vi "CH_LM Transaction.vi"(0 "Meter Index":i32, 1 "Command String":string, 3 "NofStrings (-1:all)":i32=-1, 5 "error in (no error)":errorcluster, 7 "Timeout / ms (3000)":i32=10000, 9 "Lock Timeout / ms (1000)":i32=1000) -> (11 "Lock timed out":bool, 14 "Meter Index":i32, 15 "Response":string, 17 "Response Array":string[](array[string]), 19 "error out":errorcluster)   [LabVIEW 2017, in "CH_LM.lvlib"]
doc: "This VI is used by all other VI to communicate with a LabMax. It is designed as transaction to garantee that an instruments response belongs to the causing command. A semaphore is used to implement mutual exclusion of concurrent access to the communication interface. (The semaphore is created in the CH_LM ActiveX Control.vi.)"
uses:
  CH_LM.lvlib
  CH_LM Action Enumeration.ctl
  <vilib>/Utility/error.llb/DialogType.ctl
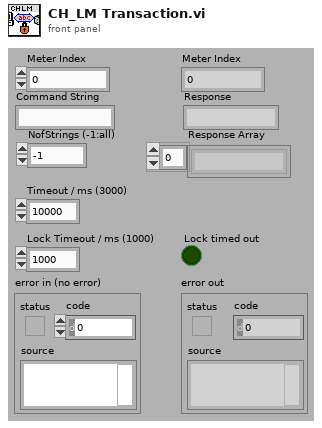
[diagram p1: front panel]
types:
  T1 = typedef "CH_LM.lvlib/CH_LM Action Enumeration.ctl" = enum16{"add", "read", "read by serial", "set", "remove", "delete", "Clear Shift-Register", ""}
  T2 = typedef "Semaphore RefNum" = refnum<k1>
  T3 = typedef "DialogType.ctl" = u16
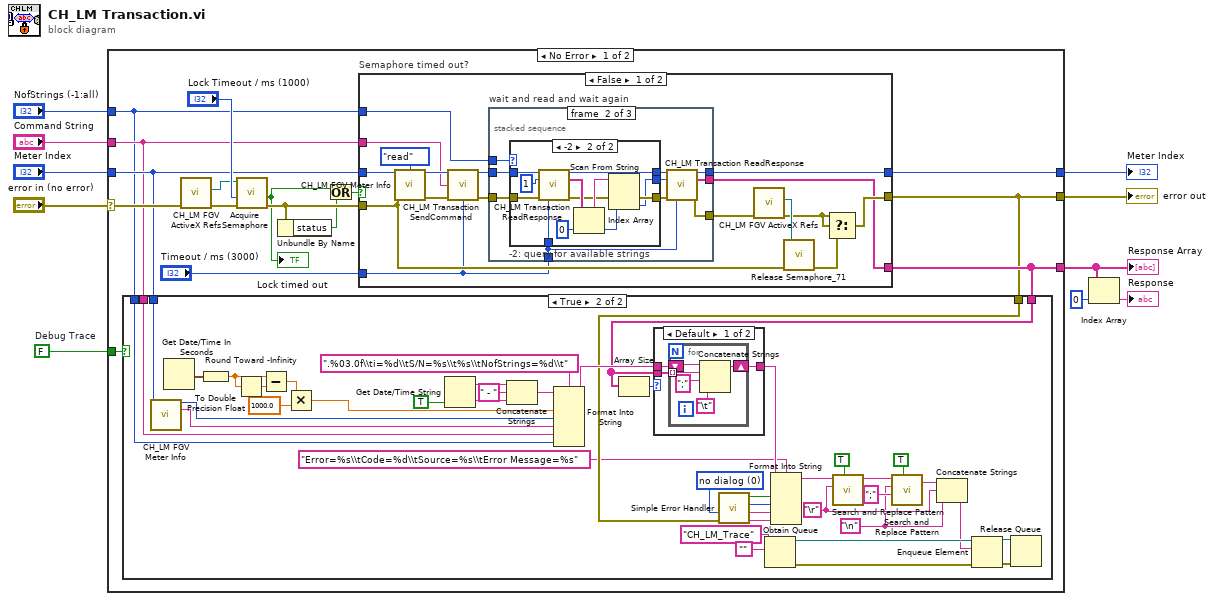
[diagram p0: block diagram]
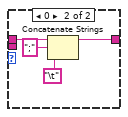
[diagram p3: hidden frame]
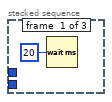
[diagram p4: hidden frame]
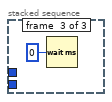
[diagram p6: hidden frame]
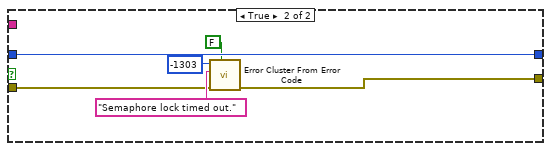
[diagram p7: hidden frame]
diagram:
  w1 = FALSE  # Debug Trace
  n1 = case shown="No Error" "error in (no error)" {
    selector: "error in (no error)" -> [w23 w132]
    tunnel: [w11 w132] -> w10
    tunnel: "Meter Index" -> [w15 w131]
    tunnel: [w12 _] -> w7
    tunnel: [w17 w131] -> w8
    tunnel: "Command String" -> [w14 _]
    tunnel: "NofStrings (-1:all)" -> [w13 _]
    tunnel: w1 -> [w16 _]
    frame No Error {
      n2 = call "CH_LM FGV ActiveX Refs.vi"("error in (no error)"=w23) -> ("error out"=w22:errorcluster, "CH_LM semaphore"=w24:T2)  [unwired: 4 in, 2 out]
      n3 = call <vilib>:"Acquire Semaphore.vi"("error in (no error)"=w22, "ms timeout (-1)"="Lock Timeout / ms (1000)", "semaphore"=w24) -> ("error out"=w21:errorcluster, "timed out"=w19:bool)  [unwired: 3 out]
      "Lock timed out" <- w19
      n4 = Unbundle By Name(w21) -> ("status"=w20:bool)
      n5 = Or(x=w19, y=w20) -> (x .or. y?=w18:bool)
      n6 = case "Semaphore timed out?" shown="False" w18 {
        tunnel: w14 -> [w92 _]
        tunnel: [w87 _] -> w12
        tunnel: [w98 w126] -> w11
        tunnel: "Timeout / ms (3000)" -> [w83 _]
        tunnel: w21 -> [w93 w127]
        tunnel: w15 -> [w95 w130]
        tunnel: w13 -> [w84 _]
        tunnel: [w88 w130] -> w17
        frame False {
          n7 = call "CH_LM FGV Meter Info.vi"("Meter Index"=w95, "Action (read)"=CH_LM_Action_Enumeration."read", "error in (no error)"=w93) -> ("Meter Index out"=w96:i32, "error out"=w94:errorcluster)  [unwired: 2 in, 9 out]
          n8 = call "CH_LM Transaction SendCommand.vi"("Meter Index"=w96, "Command String"=w92, "error in (no error)"=w94, "Timeout / ms (3000)"=w83) -> ("Meter Index out"=w85:i32, "error out"=w86:errorcluster)  [unwired: 4 in, 6 out]
          n9 = stacked-sequence "wait and read and wait again" {
            tunnel: [_ w109 _] -> w88
            tunnel: [_ w108 _] -> w87
            tunnel: w86 -> [_ w107 _]
            tunnel: w85 -> [_ w106 _]
            tunnel: w84 -> [_ w102 _]
            tunnel: w83 -> [_ w101 _]
            tunnel: [_ w100 _] -> w82
            frame #0 {
              n10 = Wait (ms)(milliseconds to wait=u32 20) -> ()  [unwired: 1 out]
            }
            frame #1 {
              n11 = case "-2: query for available strings" shown="-2" w102 {
                selector: w102 -> [w110 _]
                tunnel: w107 -> [w111 w123]
                tunnel: w106 -> [w112 w122]
                tunnel: [w112 w121] -> w105
                tunnel: [w111 w116] -> w104
                tunnel: [w110 w114] -> w103
                tunnel: w101 -> [_ w113]
                frame Default {
                }
                frame -2 {
                  w115 = 0 ("index")
                  n12 = call "CH_LM Transaction ReadResponse.vi"("Meter Index"=w122, "NofStrings (-1:all)"=1, "error in (no error)"=w123, "Timeout / ms (3000)"=w113) -> ("Meter Index out"=w121:i32, "Response Array"=w119:string[], "error out"=w117:errorcluster)  [unwired: 9 out]
                  n13 = Index Array(array=w119, index=w115) -> (element=w118:string)
                  n14 = Scan From String(input string=w118, error in=w117, default 1=w115) -> (error out=w116:errorcluster, output 1=w114:i32)  [unwired: 2 in, 2 out]
                }
              }
              n15 = call "CH_LM Transaction ReadResponse.vi"("Meter Index"=w105, "NofStrings (-1:all)"=w103, "error in (no error)"=w104, "Timeout / ms (3000)"=w101) -> ("Meter Index out"=w109:i32, "Response Array"=w108:string[], "error out"=w100:errorcluster)  [unwired: 9 out]
            }
            frame #2 {
              n16 = Wait (ms)(milliseconds to wait=u32 0) -> ()  [unwired: 1 out]
            }
          }
          n17 = call "CH_LM FGV ActiveX Refs.vi"("error in (no error)"=w82) -> ("error out"=w89:errorcluster, "CH_LM semaphore"=w90:T2)  [unwired: 4 in, 2 out]
          n18 = call <vilib>:"Release Semaphore_71.vi"("error in (no error)"=w93, "semaphore"=w90) -> ("error out"=w91:errorcluster)  [unwired: 5 out]
          n19 = Select(t=w89, s=w89, f=w91) -> (s? t:f=w98:errorcluster)
        }
        frame True {
          n20 = call <vilib>:"Error Cluster From Error Code.vi"("show call chain? (False)"=FALSE, "error in (no error)"=w127, "error message (\"\")"="Semaphore lock timed out." ("error message (\"\")"), "error code (0)"=-1303) -> ("error out"=w126:errorcluster)  [unwired: 5 out]
        }
      }
      n21 = case shown="True" w16 {
        tunnel: w14 -> [_ w57]
        tunnel: w15 -> [_ w54]
        tunnel: w12 -> [_ w36]
        tunnel: w13 -> [_ w56]
        tunnel: w11 -> [_ w45]
        frame False {
        }
        frame True {
          w38 = T3 0 items=["no dialog", "OK message", "continue or stop message", "OK message + warnings", "continue/stop + warnings"] ("type of dialog (OK msg:1)")
          w27 = "\n"
          w28 = "\r"
          n22 = call "CH_LM FGV Meter Info.vi"("Meter Index"=w54) -> ("Meter Index out"=w53:i32, "Serial Number out"=w55:string)  [unwired: 4 in, 9 out]
          n23 = Get Date/Time In Seconds() -> (seconds since 1Jan1904=w51:timestamp)
          n24 = To Double Precision Float(number=w51) -> (double precision float=w50:dbl)
          n25 = Round Toward -Infinity(1:w50) -> (0:w49:dbl)
          n26 = Subtract(x=w50, y=w49) -> (x-y=w47:dbl)
          n27 = Multiply(x=w47, y=1000.0) -> (x*y=w46:dbl)
          n28 = Get Date/Time String(want seconds? (F)=TRUE) -> (date string=w62:string, time string=w60:string)  [unwired: 2 out]
          n29 = Concatenate Strings(w62, " - " ("string"), w60) -> (w59:string)
          n30 = Format Into String(format string=".%03.0f\\ti=%d\\tS/N=%s\\t%s\\tNofStrings=%d\\t", initial string=w59, w46, w53, w55, w57, w56) -> (resulting string=w58:string)  [unwired: 1 in, 1 out]
          n31 = Array Size(array=w36) -> (size(s)=w37:i32)
          n32 = case shown="Default" w37 {
            tunnel: w36 -> [w72 _]
            tunnel: w58 -> [w71 w81]
            tunnel: [w70 w80] -> w44
            frame Default {
              n33 = for {
                tunnel: w72 -> [w76] mode=indexing
                shift-right: [w77] -> w70
                shift-left: w71 -> [w75]
                n34 = Concatenate Strings(w75, w76, ";" ("string"), "\t") -> (w77:string)
              }
            }
            frame 0 {
              n35 = Concatenate Strings(w81, ";" ("string"), "\t") -> (w80:string)
            }
          }
          n36 = call <vilib>:"Simple Error Handler.vi"("type of dialog (OK msg:1)"=w38, "error in (no error)"=w45) -> ("error?"=w43:bool, "code out"=w42:i32, "source out"=w41:string, "message"=w40:string)  [unwired: 4 out]
          n37 = Obtain Queue(name (unnamed)="CH_LM_Trace", element data type="") -> (queue out=w69:refnum<queue>, error out=w68:errorcluster)  [unwired: 3 in, 1 out]
          n38 = Format Into String(format string="Error=%s\\tCode=%d\\tSource=%s\\tError Message=%s", initial string=w44, w43, w42, w41, w40) -> (resulting string=w30:string)  [unwired: 1 in, 1 out]
          n39 = call <vilib>:"Search and Replace Pattern.vi"("string"=w30, "regular expression (\"\")"=w28, "replace all? (F)"=TRUE) -> ("result string"=w29:string)  [unwired: 1 in, 2 out]
          n40 = call <vilib>:"Search and Replace Pattern.vi"("string"=w29, "regular expression (\"\")"=w27, "replace string (\"\")"=";" ("replace string (\"\")"), "replace all? (F)"=TRUE) -> ("result string"=w33:string)  [unwired: 2 out]
          n41 = Concatenate Strings(w33, w28, w27) -> (w32:string)
          n42 = Enqueue Element(queue=w69, element=w32, error in (no error)=w68) -> (queue out=w65:refnum<queue>, error out=w64:errorcluster)  [unwired: 2 out]
          n43 = Release Queue(queue=w65, error in (no error)=w64) -> ()  [unwired: 4 out]
        }
      }
    }
    frame Error {
    }
  }
  "error out" <- w10
  "Meter Index" <- w8
  "Response Array" <- w7
  n44 = Index Array(array=w7, index=0) -> (element=→"Response":string)
